vi "Start Listener.vi"() -> ()   [LabVIEW 2014]
uses:
  Core SubVIs/Core SubVIs.lvlib
panel:
  in  "Start Matlab Script":string="z:\\users\\james\\scripts\\listener"
  in  "IP":string
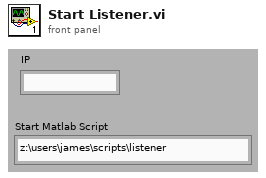
[diagram p1: front panel]
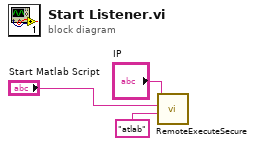
[diagram p0: block diagram]
diagram:
  n1 = call "RemoteExecuteSecure.vi"("User"="atlab", "Start Matlab Script"="Start Matlab Script", "IP"="IP") -> ()  [unwired: 9 out]
